vi "dvp Vi Set User Id.vi"(9 "pLength":u32, 10 "UserId":string, 11 "handle":u32) -> (1 "pLength out":u32, 3 "function return":u32(ring))   [LabVIEW 2018, in "LabViewDVPCamera.lvlib"]
doc: "LabviewDvp2Api dvpStatus dvpViSetUserId(dvpHandle handle, const char *UserId, dvpUint32 *pLength);"
uses:
  LabViewDVPCamera.lvlib
  LabViewDVPCamera/LabViewDVPCamera.dll
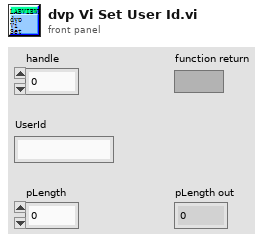
[diagram p1: front panel]
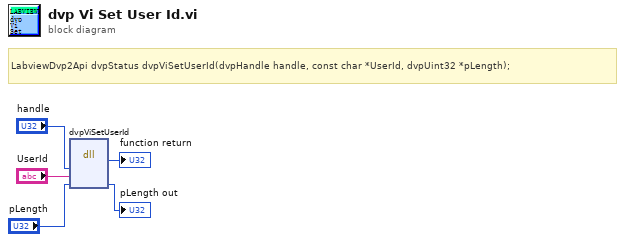
[diagram p0: block diagram]
diagram:
  # "LabviewDvp2Api dvpStatus dvpViSetUserId(dvpHandle handle, const char *UserId, dvpUint32 *pLength);"
  n1 = dll-call lib="C:/Program Files (x86)/DVP2 Labview cn 64/Sample/LabViewDVPCamera/LabViewDVPCamera.*" fn="dvpViSetUserId"("handle"="handle", "UserId"="UserId", "pLength"="pLength") -> (→"function return":u32, "pLength"=→"pLength out":u32)  [unwired: 5 in, 2 out]
